vi "SetUSB-LINK&ChkBuild-FwVer.vi"(0 "MintController":refnum<k7>(container), 11 "error in":errorcluster) -> (4 "reference out":refnum<k7>, 6 "Error?":bool, 8 "AAABuild":i32, 10 "FirmwareVersion":string, 15 "error out":errorcluster)   [LabVIEW 2011]
panel:
  out "error AAABuild":errorcluster
  out "error SetUSBlink":errorcluster
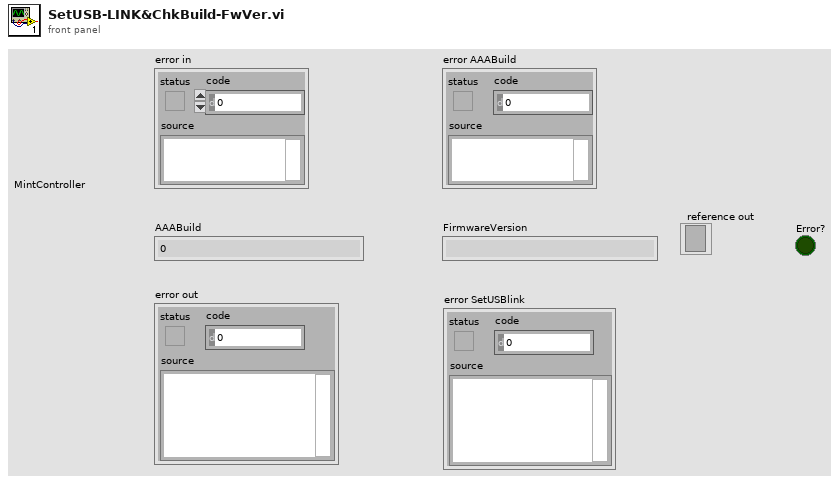
[diagram p1: front panel]
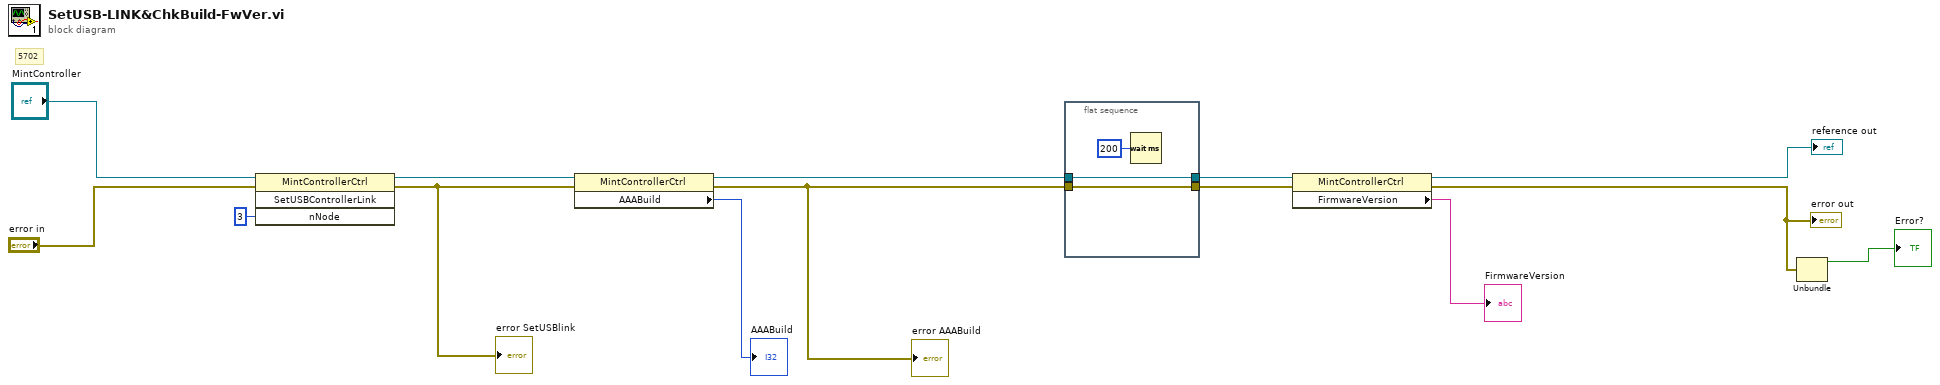
[diagram p0: block diagram]
diagram:
  # "5702"
  n1 = invoke class="MintControllerCtrl" method="SetUSBControllerLink"(reference="MintController", error in="error in", "nNode"=i16 3) -> (reference out=w2:refnum<k7>, error out=w1:errorcluster)  [unwired: 1 in, 2 out]
  "error SetUSBlink" <- w1
  n2 = property class="MintControllerCtrl"(reference=w2, error in=w1) -> (reference out=w8:refnum<k7>, error out=w7:errorcluster, "AAABuild"=→"AAABuild":i32)
  "error AAABuild" <- w7
  n3 = flat-sequence {
    tunnel: w8 -> [w16]
    tunnel: w7 -> [w15]
    tunnel: [w16] -> w6
    tunnel: [w15] -> w5
    frame #0 {
      n4 = Wait (ms)(milliseconds to wait=u32 200) -> ()  [unwired: 1 out]
    }
  }
  n5 = property class="MintControllerCtrl"(reference=w6, error in=w5) -> (reference out=→"reference out":refnum<k7>, error out=w11:errorcluster, "FirmwareVersion"=→"FirmwareVersion":string)
  "error out" <- w11
  n6 = Unbundle(w11) -> ("status"=→"Error?":bool)  [unwired: 2 out]
